vi "Grab from Camera.vi"(3 "Error":string, 5 "Image":T1={"Image ID"=0, "Channel ID"=-1}) -> (0 "Error":string, 1 "Millisecond time":u32, 2 "Image":T1={"Image ID"=0, "Channel ID"=-1})   [LabVIEW 2011, in "labvvis.lvlib"]
doc: "Copies a single frame from the first available sequence grabber to Image.\n\nMillisecond time returns the time that the frame was captured.\n\nImage should be either a RGBA or grey-scale image of the size specified by Camera Image Size."
uses:
  <userlib>/labvvis/labvvis.lvlib
  labvvis.framework
  <userlib>/labvvis/VVIS Image.ctl
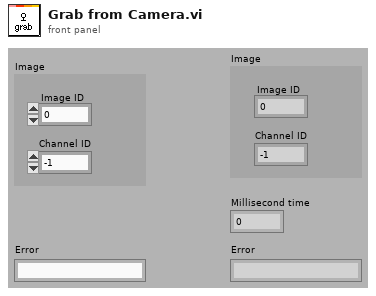
[diagram p1: front panel]
types:
  T1 = typedef "labvvis.lvlib/VVIS Image.ctl" = cluster{"Image ID":i16, "Channel ID":i16}
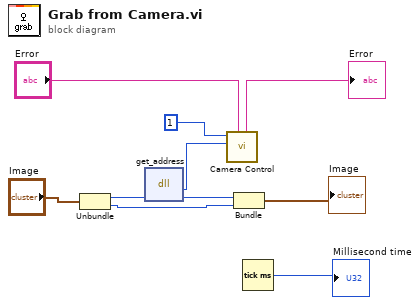
[diagram p0: block diagram]
diagram:
  n1 = Unbundle("Image") -> ("Image ID"=w9:i16, "Channel ID"=w1:i16)
  n2 = dll-call lib="labvvis.framework" fn="get_address"("image_id"=w9) -> (w6:i32, "image_id"=w8:i16)  [unwired: 3 in, 2 out]
  n3 = call <userlib>:"Camera Control.vi"("Error"="Error", "Image Pointer"=w6, "Operation"=i8 1) -> ("Error"=→"Error":string)  [unwired: 2 in, 4 out]
  n4 = Bundle("image_id"=w8, "Channel ID"=w1) -> (→"Image":cluster{"image_id":i16, "Channel ID":i16})  [unwired: 1 in]
  n5 = Tick Count (ms)() -> (millisecond timer value=→"Millisecond time":u32)
